vi "Start CSM DebugTool Dialog.vi"(8 "error in (no error)":errorcluster, 11 "Application In":refnum<vi>) -> (0 "error out":errorcluster)   [LabVIEW 2017, in "CSM DebugTool Dialog.lvlib"]
uses:
  CSM DebugTool Dialog.lvlib
  _Shared/CSM Shared.lvlib
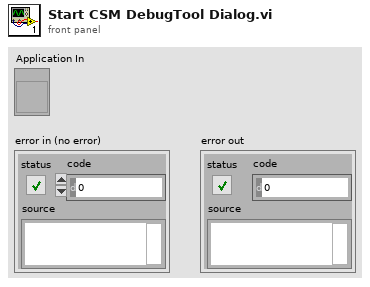
[diagram p1: front panel]
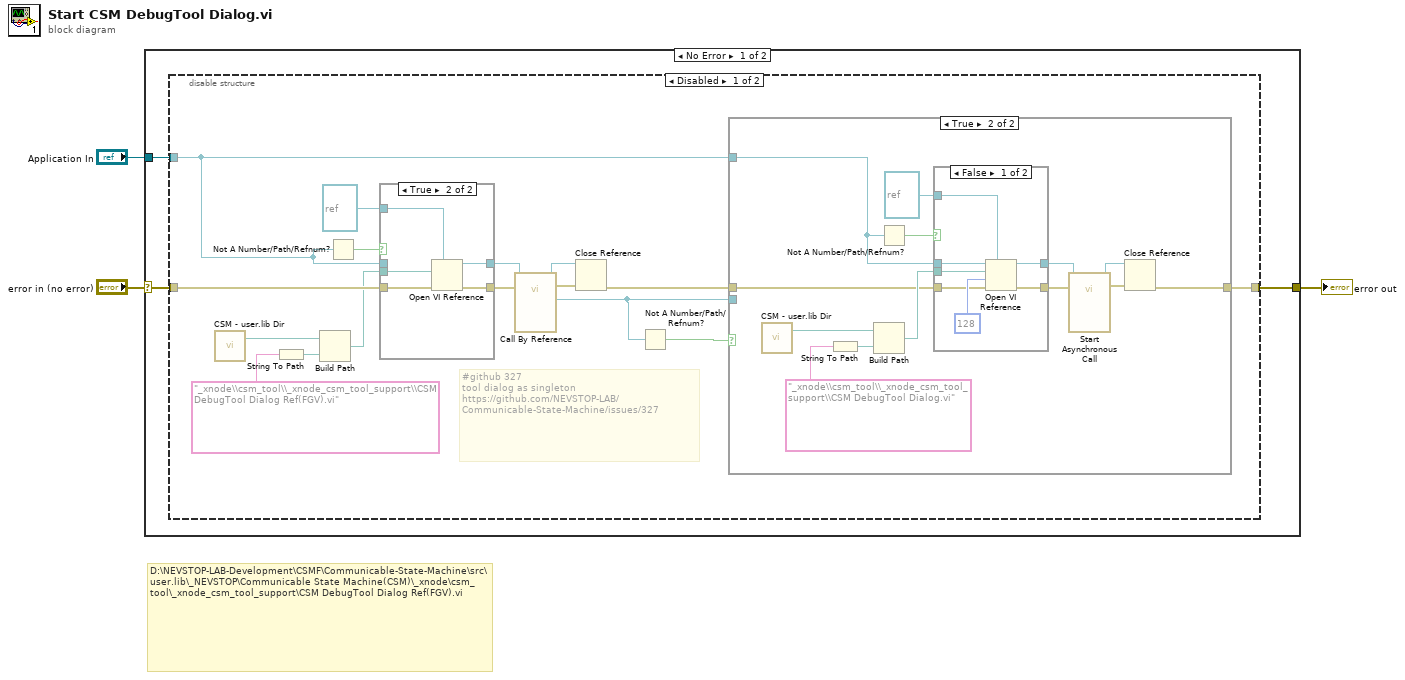
[diagram p0: block diagram]
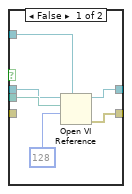
[diagram p2: hidden frame]
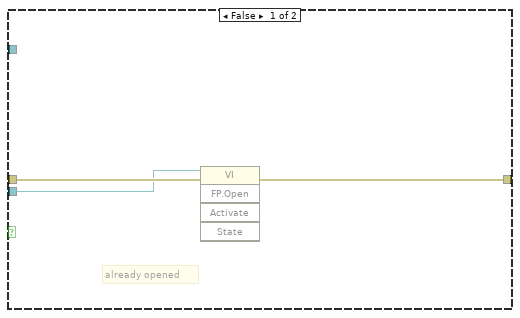
[diagram p3: hidden frame]
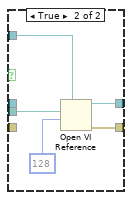
[diagram p4: hidden frame]
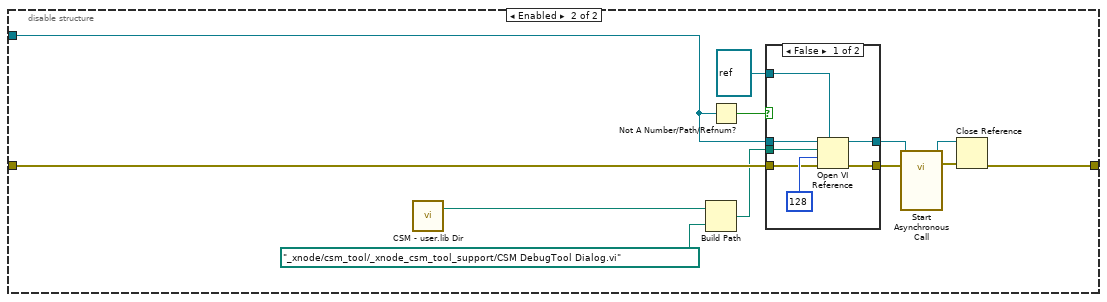
[diagram p5: hidden frame]
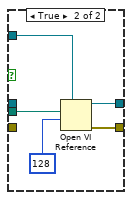
[diagram p6: hidden frame]
diagram:
  # "D:\\NEVSTOP-LAB-Development\\CSMF\\Communicable-State-Machine\\src\\user.lib\\_NEVSTOP\\Communicable State Machine(CSM)\\_xnode\\csm_tool\\_xnode_csm_tool_support\\CSM DebugTool Dialog Ref(FGV).vi"
  n1 = case shown="No Error" "error in (no error)" {
    selector: "error in (no error)" -> [w5 w86]
    tunnel: [w6 w86] -> w3
    tunnel: "Application In" -> [w4 _]
    frame No Error {
      n2 = disable-structure shown="Disabled" {
        disable-tunnel: [w22 w73] -> w6
        disable-tunnel: w5 -> [w21 w72]
        disable-tunnel: w4 -> [w19 w71]
        frame Disabled {
          # "#github 327 \ntool dialog as singleton\nhttps://github.com/NEVSTOP-LAB/Communicable-State-Machine/issues/327"
          n3 = call "CSM - user.lib Dir.vi"() -> ("csm_user.lib_dir"=w11:path)  [unwired: 2 in, 1 out]
          n4 = String To Path(string="_xnode\\csm_tool\\_xnode_csm_tool_support\\CSM DebugTool Dialog Ref(FGV).vi" ("name or relative path")) -> (path=w7:path)
          n5 = Build Path(base path=w11, name or relative path=w7) -> (appended path=w12:path)
          n6 = Not A Number/Path/Refnum?(number/path/refnum=w19) -> (NaN/Path/Refnum?=w10:bool)
          n7 = case shown="True" w10 {
            tunnel: [w28 w33] -> w14
            tunnel: [w27 w32] -> w13
            tunnel: w12 -> [w26 w31]
            tunnel: w19 -> [w24 _]
            tunnel: refnum<vi> refnum ("type specifier VI Refnum (for type only)") -> [w23 w30]
            tunnel: w21 -> [_ w29]
            frame False {
              n8 = Open VI Reference(type specifier VI Refnum (for type only)=w23, application reference (local)=w24, vi path=w26, options=128) -> (vi reference=w28:refnum<vi>, error out=w27:errorcluster)  [unwired: 2 in]
            }
            frame True {
              n9 = Open VI Reference(type specifier VI Refnum (for type only)=w30, vi path=w31, error in (no error)=w29) -> (vi reference=w33:refnum<vi>, error out=w32:errorcluster)  [unwired: 3 in]
            }
          }
          n10 = call-by-ref "?"(reference=w14, error in=w13) -> (reference out=w16:refnum<vi>, error out=w15:errorcluster, "VI Reference(out)"=w17:refnum<vi>)  [unwired: 11 in]
          n11 = Close Reference(reference=w16, error in (no error)=w15) -> (error out=w18:errorcluster)
          n12 = Not A Number/Path/Refnum?(number/path/refnum=w17) -> (NaN/Path/Refnum?=w20:bool)
          n13 = case shown="True" w20 {
            tunnel: [w36 w42] -> w22
            tunnel: w19 -> [_ w40]
            tunnel: w18 -> [w35 w38]
            tunnel: w17 -> [w34 _]
            frame False {
              # "already opened"
              n14 = invoke class="VI" method="FP.Open"(reference=w34, error in=w35) -> (error out=w36:errorcluster)  [unwired: 3 in, 4 out]
            }
            frame True {
              n15 = call "CSM - user.lib Dir.vi"() -> ("csm_user.lib_dir"=w43:path)  [unwired: 2 in, 1 out]
              n16 = String To Path(string="_xnode\\csm_tool\\_xnode_csm_tool_support\\CSM DebugTool Dialog.vi" ("name or relative path")) -> (path=w37:path)
              n17 = Build Path(base path=w43, name or relative path=w37) -> (appended path=w44:path)
              n18 = Not A Number/Path/Refnum?(number/path/refnum=w40) -> (NaN/Path/Refnum?=w41:bool)
              n19 = case shown="False" w41 {
                tunnel: [w56 w61] -> w46
                tunnel: [w55 w60] -> w45
                tunnel: w44 -> [w54 w59]
                tunnel: w40 -> [w52 _]
                tunnel: refnum<vi> refnum ("type specifier VI Refnum (for type only)") -> [w51 w57]
                tunnel: w38 -> [w50 _]
                frame False {
                  n20 = Open VI Reference(type specifier VI Refnum (for type only)=w51, application reference (local)=w52, vi path=w54, options=128, error in (no error)=w50) -> (vi reference=w56:refnum<vi>, error out=w55:errorcluster)  [unwired: 1 in]
                }
                frame True {
                  n21 = Open VI Reference(type specifier VI Refnum (for type only)=w57, vi path=w59, options=128) -> (vi reference=w61:refnum<vi>, error out=w60:errorcluster)  [unwired: 3 in]
                }
              }
              n22 = call-by-ref "Start Asynchronous Call"(reference=w46, error in=w45) -> (reference out=w48:refnum<vi>, error out=w47:errorcluster)  [unwired: 12 in]
              n23 = Close Reference(reference=w48, error in (no error)=w47) -> (error out=w42:errorcluster)
            }
          }
        }
        frame Enabled {
          n24 = call "CSM - user.lib Dir.vi"() -> ("csm_user.lib_dir"=w65:path)  [unwired: 2 in, 1 out]
          n25 = Build Path(base path=w65, name or relative path=path "_xnode/csm_tool/_xnode_csm_tool_support/CSM DebugTool Dialog.vi") -> (appended path=w66:path)
          n26 = Not A Number/Path/Refnum?(number/path/refnum=w71) -> (NaN/Path/Refnum?=w64:bool)
          n27 = case shown="False" w64 {
            tunnel: [w80 w85] -> w68
            tunnel: [w79 w84] -> w67
            tunnel: w66 -> [w78 w83]
            tunnel: w71 -> [w76 _]
            tunnel: refnum<vi> refnum ("type specifier VI Refnum (for type only)") -> [w75 w81]
            tunnel: w72 -> [w74 _]
            frame False {
              n28 = Open VI Reference(type specifier VI Refnum (for type only)=w75, application reference (local)=w76, vi path=w78, options=128, error in (no error)=w74) -> (vi reference=w80:refnum<vi>, error out=w79:errorcluster)  [unwired: 1 in]
            }
            frame True {
              n29 = Open VI Reference(type specifier VI Refnum (for type only)=w81, vi path=w83, options=128) -> (vi reference=w85:refnum<vi>, error out=w84:errorcluster)  [unwired: 3 in]
            }
          }
          n30 = call-by-ref "Start Asynchronous Call"(reference=w68, error in=w67) -> (reference out=w70:refnum<vi>, error out=w69:errorcluster)  [unwired: 12 in]
          n31 = Close Reference(reference=w70, error in (no error)=w69) -> (error out=w73:errorcluster)
        }
      }
    }
    frame Error {
    }
  }
  "error out" <- w3
